vi "LVClass_WavefrontCorrector Set Temporization.vi"(0 "WavefrontCorrector in":refnum<class "WavefrontCorrector.lvclass">, 5 "Sleep after command apply (ms)":i32, 11 "error in (no error)":errorcluster) -> (4 "WavefrontCorrector out":refnum<class "WavefrontCorrector.lvclass">, 15 "error out":errorcluster)   [LabVIEW 2020, in "WavefrontCorrector.lvclass"]
doc: "<B>correctorIn</B> : WavefrontCorrector object.\n<B>correctorOut</B> : WavefrontCorrector object.\n<B>sleep_after_movement</B> : WavefrontCorrector preferences : Time to stabilization (ms)."
uses:
  WavefrontCorrector.lvclass
  WavefrontCorrector.lvclass/WavefrontCorrector.ctl
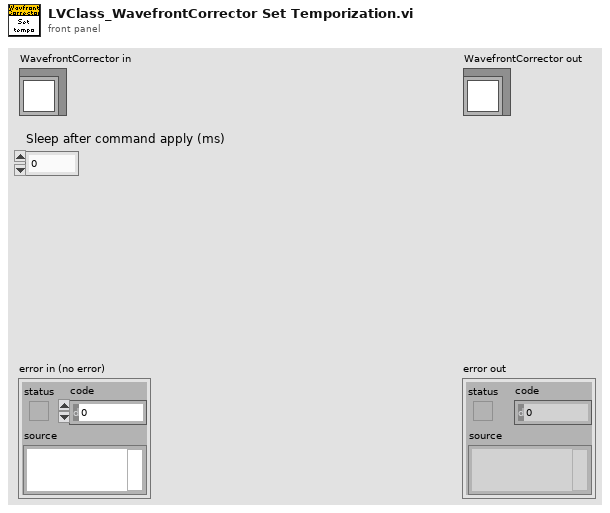
[diagram p1: front panel]
types:
  T1 = typedef "ClassID.ctl" = i64
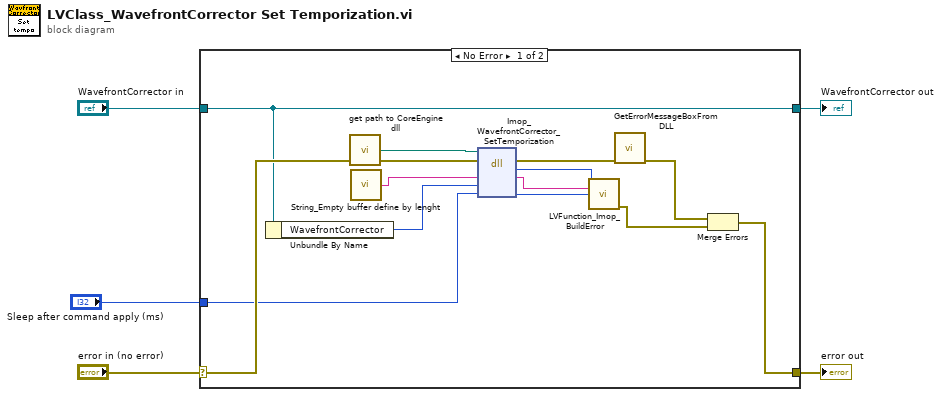
[diagram p0: block diagram]
diagram:
  n1 = case shown="No Error" "error in (no error)" {
    selector: "error in (no error)" -> [w16 w20]
    tunnel: [w7 w20] -> w4
    tunnel: [w15 w19] -> w2
    tunnel: "WavefrontCorrector in" -> [w15 w19]
    tunnel: "Sleep after command apply (ms)" -> [w13 _]
    frame No Error {
      n2 = Unbundle By Name(w15) -> ("WavefrontCorrector"=w14:T1)
      n3 = call "get path to CoreEngine dll.vi"() -> ("path to wavekit library"=w18:path)  [unwired: 14 in, 1 out]
      n4 = call "String_Empty buffer define by lenght.vi"() -> ("Empty buffer"=w17:string)  [unwired: 1 in]
      n5 = dll-call lib="D:/FLE/0.Code/CoreEngine4_Suite/LV2011_interface/DLLs/c_interface_vc100.dll" fn="Imop_WavefrontCorrector_SetTemporization"(path in=w18, error in=w16, "message"=w17, "WavefrontCorrector"=w14, "Sleep after movement"=w13) -> (error out=w10:errorcluster, "return type"=w12:i32, "message"=w11:string, "WavefrontCorrector"=w6:i64)  [unwired: 2 in, 1 out]
      n6 = call "LVFunction_Imop_BuildError.vi"("code"=w12, "String to Prepend to source (\"\")"=w11, "Adresse"=w6) -> ("error out"=w8:errorcluster)  [unwired: 12 in]
      n7 = call "GetErrorMessageBoxFromDLL.vi"("error IN"=w10) -> ("error OUT"=w9:errorcluster)  [unwired: 10 in]
      n8 = Merge Errors(w9, w8) -> (w7:errorcluster)
    }
    frame Error {
    }
  }
  "error out" <- w4
  "WavefrontCorrector out" <- w2
